vi "Test 2.vi"(8 "error in (no error)":errorcluster, 11 "Test Case In":refnum<class "Tests.lvclass">) -> (0 "error out":errorcluster, 3 "Test Case Out":refnum<class "Tests.lvclass">)   [LabVIEW 2021, in "Tests.lvclass"]
uses:
  Tests.lvclass
  C:/Program Files (x86)/National Instruments/LabVIEW 2021/vi.lib/Astemes/LUnit/Test Case.lvclass
  <vilib>/Astemes/LUnit/Test Case.lvclass/Test Case.ctl
  4993e8ee-a06a-463a-9684-69129f64d5ce.vi
  <vilib>/Astemes/LUnit/Append Pass Result.vi
  <vilib>/Astemes/LUnit/Append Fail Result.vi
  <vilib>/Astemes/LUnit/Compare Variants.vi
  <vilib>/Astemes/LUnit/Describe Comparison of Arrays.vi
  <vilib>/Astemes/LUnit/Variant to string.vi
  <vilib>/AdvancedString/1D String Array to Delimited String.vi
  <vilib>/Utility/Data Type/Get Type Information.vi
  <vilib>/Utility/LVClass/Get LV Class Name.vi
  Proto/Maze.lvclass
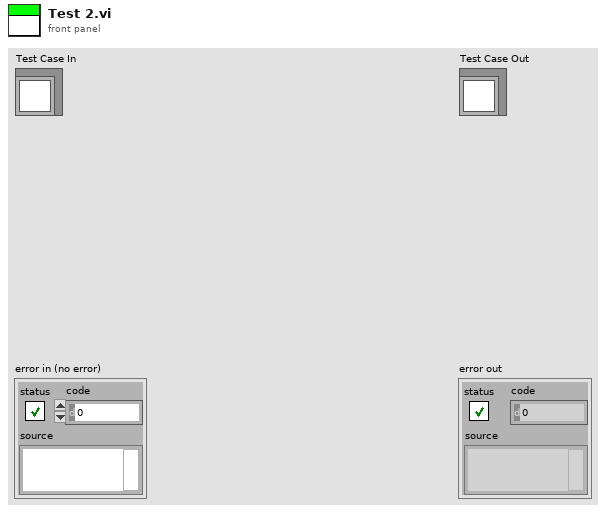
[diagram p1: front panel]
types:
  T1 = cluster{"row":i32, "col":i32, "Arriving from":enum16{"North", "South", "East", "West"}}
  T2 = cluster{"row":i32, "col":i32, "Arriving from":enum16{"North", "South", "East", "West"}}[]
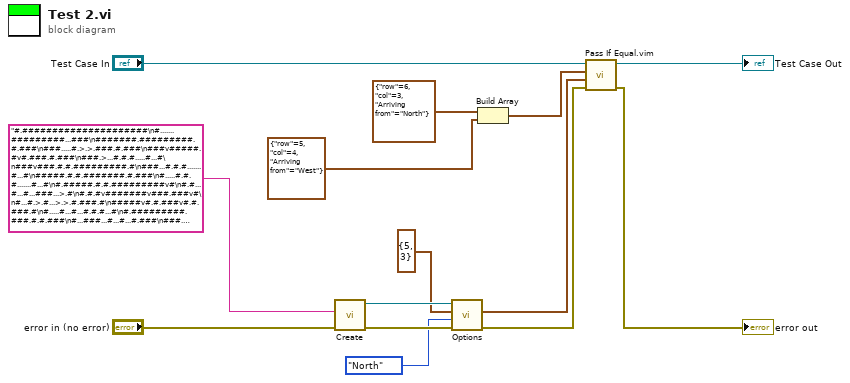
[diagram p0: block diagram]
diagram:
  n1 = call "Create.vi"("error in (no error)"="error in (no error)", "Input"="#.#####################\n#.......#########...###\n#######.#########.#.###\n###.....#.>.>.###.#.###\n###v#####.#v#.###.#.###\n###.>...#.#.#.....#...#\n###v###.#.#.#########.#\n###...#.#.#.......#...#\n#####.#.#.#######.#.###\n#.....#.#.#.......#...#\n#.#####.#.#.#########v#\n#.#...#...#...###...>.#\n#.#.#v#######v###.###v#\n#...#.>.#...>.>.#.###.#\n#####v#.#.###v#.#.###.#\n#.....#...#...#.#.#...#\n#.#########.###.#.#.###\n#...###...#...#...#.###\n###.###.#.###v#####v###\n#...#...#.#.>.>.#.>.###\n#.###.###.#.###.#.#v###\n#.....###...###...#...#\n#####################.#") -> ("error out"=w10:errorcluster, "Proto"=w8:refnum<class "Maze.lvclass">)  [unwired: 8 in]
  n2 = call "Options.vi"("error in (no error)"=w10, "Arriving from"=enum16{"North", "South", "East", "West"}."North", "Cluster"=cluster{"row":i32, "col":i32} {"row"=5, "col"=3}, "Maze In"=w8) -> ("error out"=w9:errorcluster, "Possible Steps"=w4:T2)  [unwired: 5 in, 1 out]
  n3 = Build Array(T1 {"row"=6, "col"=3, "Arriving from"=enum."North"} ("Cluster"), T1 {"row"=5, "col"=4, "Arriving from"=enum."West"} ("Cluster")) -> (w2:T2)
  n4 = call "Pass If Equal.vim"("error in (no error)"=w9, "Actual"=w4, "Expected"=w2, "LUnit Test Case In"="Test Case In") -> ("error out"=→"error out":errorcluster, "LUnit Test Case Out"=→"Test Case Out":refnum<class "Tests.lvclass">)  [unwired: 6 in]
